vi "distanceBallToOurGoalie.vi"(8 "error in (no error)":errorcluster, 10 "Game":refnum<class "Game.lvclass">, 11 "Utilities in":refnum<class "Utilities.lvclass">) -> (0 "error out":errorcluster, 2 "Robot":refnum<class "Robot.lvclass">, 3 "Utilities out":refnum<class "Utilities.lvclass">)   [LabVIEW 2023, in "Utilities.lvclass"]
uses:
  Utilities.lvclass
  Game_class/Game.lvclass
  Robot_class/Robot.lvclass
  Game_class/Game.lvclass/Game.ctl
  Team_class/Team.lvclass/Team.ctl
  Referee_class/Referee.lvclass/Referee.ctl
  Robot_class/Robot.lvclass/Robot.ctl
  Robot_class/Read id.vi
  Game_class/Read Referee.vi
  Referee_class/Read our_goalie_id.vi
  Game_class/Read AllyRef.vi
  Team_class/Read RobotRef.vi
  Ally_class/Ally.lvclass
  C:/Users/roboi/Downloads/VSS_AI-Larc2023/Team_class/Team.lvclass
  Referee_class/Referee.lvclass
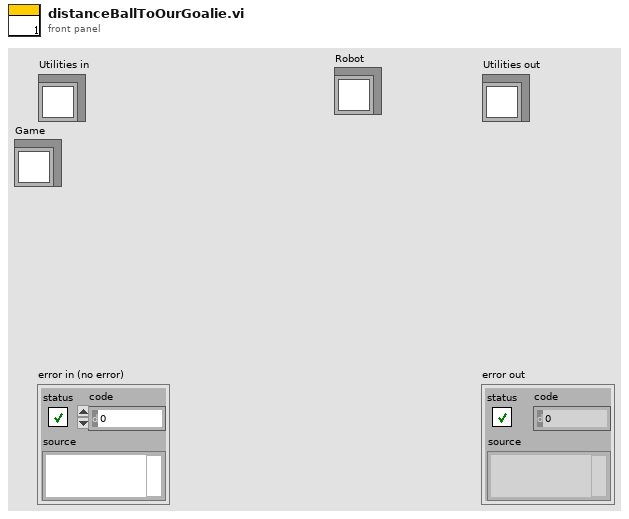
[diagram p1: front panel]
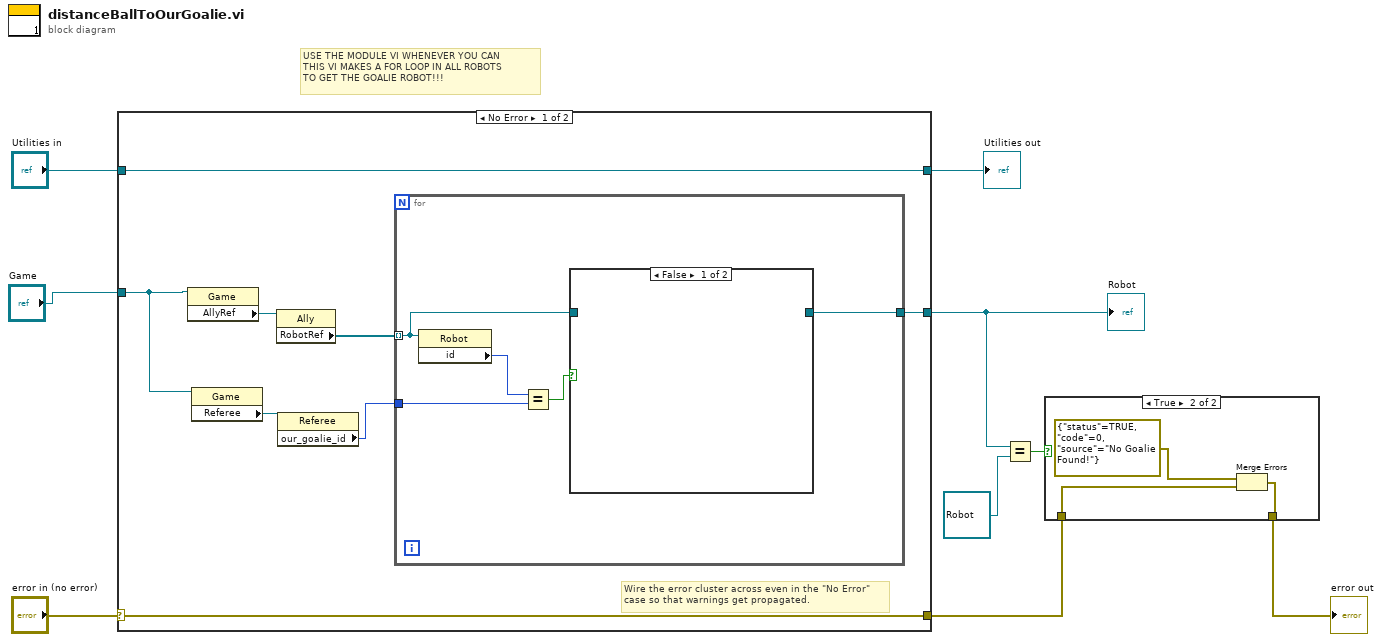
[diagram p0: block diagram]
diagram:
  # "USE THE MODULE VI WHENEVER YOU CAN\nTHIS VI MAKES A FOR LOOP IN ALL ROBOTS \nTO GET THE GOALIE ROBOT!!!"
  n1 = case shown="No Error" "error in (no error)" {
    selector: "error in (no error)" -> [w16 w25]
    tunnel: [w16 w25] -> w2
    tunnel: [w17 w24] -> w7
    tunnel: "Utilities in" -> [w17 w24]
    tunnel: "Game" -> [w13 _]
    tunnel: [w10 _] -> w4
    frame No Error {
      # "Wire the error cluster across even in the \"No Error\"\ncase so that warnings get propagated."
      n2 = property class="Game"(reference=w13) -> ("AllyRef"=w15:refnum<class "Ally.lvclass">)  [unwired: 1 in, 2 out]
      n3 = property class="Game"(reference=w13) -> ("Referee"=w12:refnum<class "Referee.lvclass">)  [unwired: 1 in, 2 out]
      n4 = property class="Ally"(reference=w15) -> ("RobotRef"=w14:refnum<class "Robot.lvclass">[])  [unwired: 1 in, 2 out]
      n5 = property class="Referee"(reference=w12) -> ("our_goalie_id"=w11:i32)  [unwired: 1 in, 2 out]
      n6 = for {
        tunnel: w14 -> [w18] mode=indexing
        tunnel: w11 -> [w22]
        tunnel: [w19] -> w10
        n7 = property class="Robot"(reference=w18) -> ("id"=w21:i32)  [unwired: 1 in, 2 out]
        n8 = Equal?(x=w21, y=w22) -> (x = y?=w20:bool)
        n9 = case shown="False" w20 {
          tunnel: [_ w23] -> w19
          tunnel: w18 -> [_ w23]
          frame False {
          }
          frame True {
          }
        }
      }
    }
    frame Error {
    }
  }
  "Utilities out" <- w7
  "Robot" <- w4
  n10 = Equal?(x=w4, y=refnum<class "Robot.lvclass"> refnum ("Robot")) -> (x = y?=w5:bool)
  n11 = case shown="True" w5 {
    tunnel: w2 -> [w26 w29]
    tunnel: [w26 w28] -> w1
    frame False {
    }
    frame True {
      n12 = Merge Errors(errorcluster {"status"=TRUE, "code"=0, "source"="No Goalie Found!"} ("error constant"), w29) -> (w28:errorcluster)
    }
  }
  "error out" <- w1
